vi "Quick Print VI or Documentation.vi"(6 "custom contents options":T13 {"list of controls options"."list which controls?" items=["all controls", "connected controls"]}, 7 "layout options":T1={"orientation (unchanged)"=0, "panel scaling for page (unchanged)"=0, "margins"={"override VI margins (false)"=FALSE, "margins (1.00)"={"top"=1.0, "left"=1.0, "right"=1.0, "bottom"=1.0}, "measurement system (default)"=0}, "printer options"={"destination printer name (current)"="", "printing method (unchanged)"=0, "color or monochrome (unchanged)"=0}, "page header options"={"page headers (unchanged)"=0, "page header content options"={"Include VI Name"=TRUE, "Include VI Path"=TRUE, "Include Last Modification Date"=TRUE, "Include Date Printed"=TRUE, "Include Page Number"=TRUE, "Include VI Icon"=TRUE}}} {"page header options"."page headers (unchanged)" items=["Unchanged", "Include page headers", "Do not include page headers"]; "printer options"."color or monochrome (unchanged)" items=["Unchanged", "Color/grayscale", "Monochrome"]; "printer options"."printing method (unchanged)" items=["Unchanged", "Standard", "PostScript", "Bitmap"]; "panel scaling for page (unchanged)" items=["Unchanged", "No Scaling", "Scale front panel to fit"]; "orientation (unchanged)" items=["Unchanged", "portrait", "landscape"]; "margins"."measurement system (default)" items=["Default", "US", "Metric"]; "margins"."margins (1.00)"."right" format="%.2f"; "margins"."margins (1.00)"."bottom" format="%.2f"; "margins"."margins (1.00)"."top" format="%.2f"; "margins"."margins (1.00)"."left" format="%.2f"}, 8 "error in (no error)":errorcluster, 10 "contents (complete front panel)":T15 items=["Complete front panel", "Visible portion of front panel", "Icon, description, panel and diagram", "Documentation: Using the panel", "Documentation: Using as a subVI", "Documentation: Complete", "Documentation: Custom"], 11 "VI reference":refnum<vi>) -> (0 "error out":errorcluster)   [LabVIEW 2020, in "NI_ReportGenerationCore.lvlib"]
uses:
  <vilib>/Utility/NIReport.llb/NI_ReportGenerationCore.lvlib
  <vilib>/printing/EasyPrintingControls.llb/contents.ctl
  <vilib>/printing/EasyPrintingControls.llb/custom_contents_options.ctl
  <vilib>/printing/EasyPrintingControls.llb/list_which_controls.ctl
  <vilib>/printing/EasyPrintingControls.llb/layout_options.ctl
  <vilib>/printing/EasyPrintingControls.llb/orientation.ctl
  <vilib>/printing/EasyPrintingControls.llb/panel_scaling_for_page.ctl
  <vilib>/printing/EasyPrintingControls.llb/margins.ctl
  <vilib>/printing/EasyPrintingControls.llb/margin_values.ctl
  <vilib>/printing/EasyPrintingControls.llb/measurement_system.ctl
  <vilib>/printing/EasyPrintingControls.llb/printer_options.ctl
  <vilib>/printing/EasyPrintingControls.llb/printing_method.ctl
  <vilib>/printing/EasyPrintingControls.llb/color_or_monochrome.ctl
  <vilib>/printing/EasyPrintingControls.llb/page_header_options.ctl
  <vilib>/printing/EasyPrintingControls.llb/page_headers.ctl
  <vilib>/printing/EasyPrintingControls.llb/page_header_content_options.ctl
  <vilib>/printing/EasyPrintingControls.llb/contents_ENUM.ctl
panel:
  in  "VI Type Names":string[](array[string])=["invalid VI type", "Standard VI", "Control VI", "Global VI", "Polymorphic VI"]
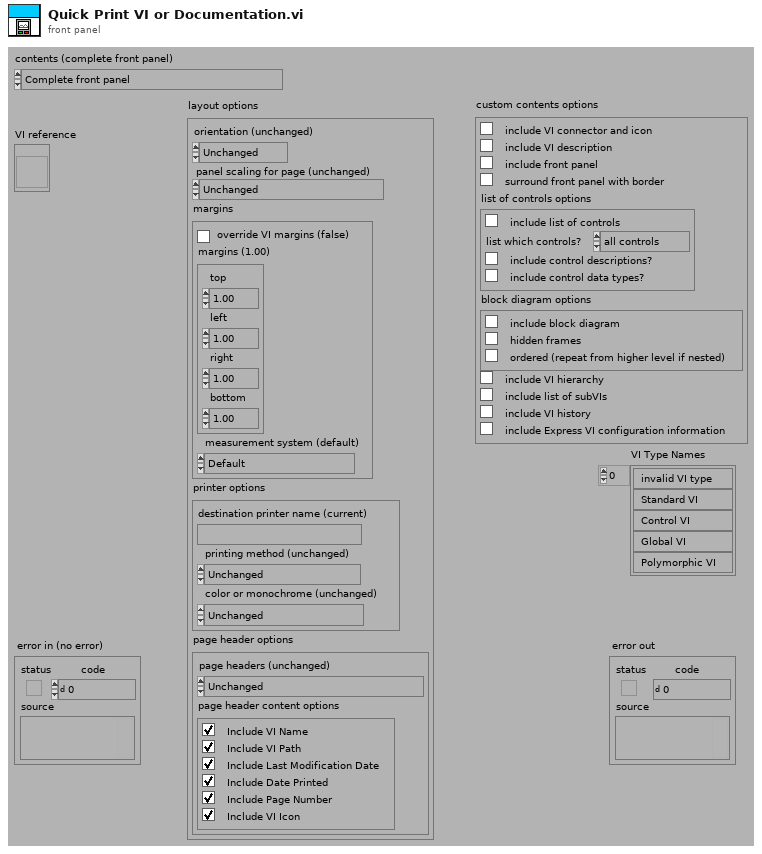
[diagram p1: front panel]
types:
  T1 = typedef "NI_ReportGenerationCore.lvlib/layout_options.ctl" = cluster{"orientation (unchanged)":T2, "panel scaling for page (unchanged)":T3, "margins":T4, "printer options":T7, "page header options":T10}
  T2 = typedef "NI_ReportGenerationCore.lvlib/orientation.ctl" = u16
  T3 = typedef "NI_ReportGenerationCore.lvlib/panel_scaling_for_page.ctl" = u16
  T4 = typedef "NI_ReportGenerationCore.lvlib/margins.ctl" = cluster{"override VI margins (false)":bool, "margins (1.00)":T5, "measurement system (default)":T6}
  T5 = typedef "NI_ReportGenerationCore.lvlib/margin_values.ctl" = cluster{"top":dbl, "left":dbl, "right":dbl, "bottom":dbl}
  T6 = typedef "NI_ReportGenerationCore.lvlib/measurement_system.ctl" = u16
  T7 = typedef "NI_ReportGenerationCore.lvlib/printer_options.ctl" = cluster{"destination printer name (current)":string, "printing method (unchanged)":T8, "color or monochrome (unchanged)":T9}
  T8 = typedef "NI_ReportGenerationCore.lvlib/printing_method.ctl" = u16
  T9 = typedef "NI_ReportGenerationCore.lvlib/color_or_monochrome.ctl" = u16
  T10 = typedef "NI_ReportGenerationCore.lvlib/page_header_options.ctl" = cluster{"page headers (unchanged)":T11, "page header content options":T12}
  T11 = typedef "NI_ReportGenerationCore.lvlib/page_headers.ctl" = u16
  T12 = typedef "NI_ReportGenerationCore.lvlib/page_header_content_options.ctl" = cluster{"Include VI Name":bool, "Include VI Path":bool, "Include Last Modification Date":bool, "Include Date Printed":bool, "Include Page Number":bool, "Include VI Icon":bool}
  T13 = typedef "NI_ReportGenerationCore.lvlib/custom_contents_options.ctl" = cluster{"include VI connector and icon":bool, "include VI description":bool, "include front panel":bool, "surround front panel with border":bool, "list of controls options":cluster{"include list of controls":bool, "list which controls?":T14, "include control descriptions?":bool, "include control data types?":bool}, "block diagram options":cluster{"include block diagram":bool, "hidden frames":bool, "ordered (repeat from higher level if nested)":bool}, "include VI hierarchy":bool, "include list of subVIs":bool, "include VI history":bool, "include Express VI configuration information":bool}
  T14 = typedef "NI_ReportGenerationCore.lvlib/list_which_controls.ctl" = u16
  T15 = typedef "NI_ReportGenerationCore.lvlib/contents.ctl" = u16
  T16 = typedef "NI_ReportGenerationCore.lvlib/contents_ENUM.ctl" = enum16{"Complete front panel", "Visible portion of front panel", "Icon, description, panel and diagram", "Documentation: Using the panel", "Documentation: Using as a subVI", "Documentation: Complete", "Documentation: Custom"}
  T17 = enum32{"invalid VI type", "Standard VI", "Control VI", "Global VI", "Polymorphic VI", "Configuration VI", "SubSystem", "Facade VI", "Method VI", "Statechart Diagram VI"}
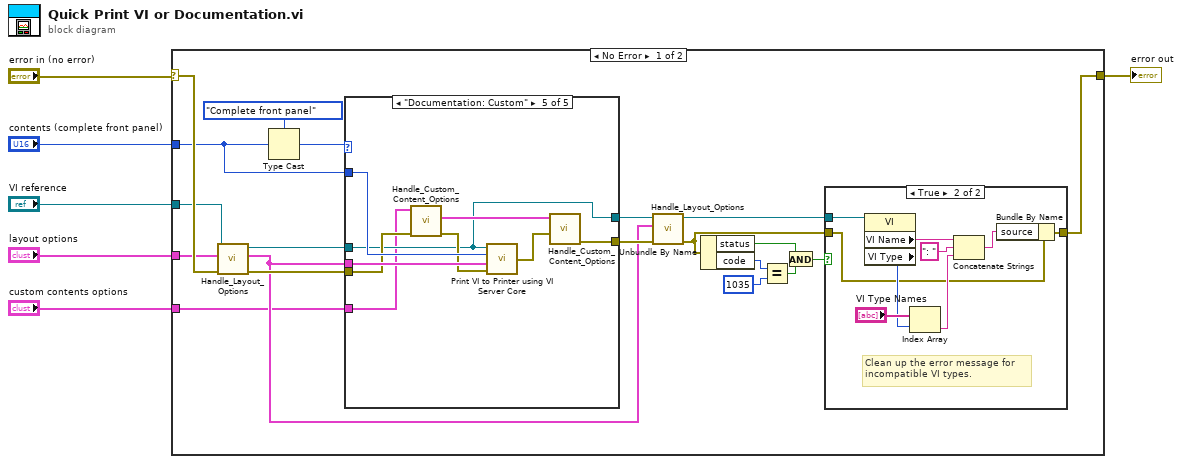
[diagram p0: block diagram]
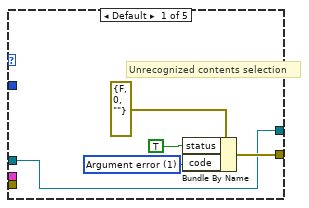
[diagram p3: hidden frame]
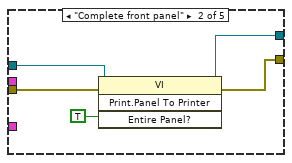
[diagram p4: hidden frame]
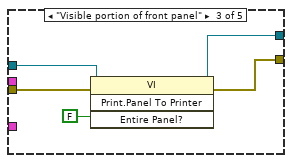
[diagram p5: hidden frame]
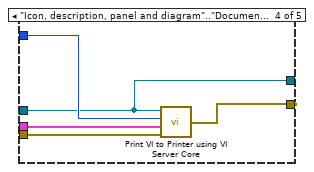
[diagram p6: hidden frame]
diagram:
  n1 = case shown="No Error" "error in (no error)" {
    selector: "error in (no error)" -> [w26 w66]
    tunnel: [w11 w66] -> w5
    tunnel: "contents (complete front panel)" -> [w10 _]
    tunnel: "layout options" -> [w9 _]
    tunnel: "custom contents options" -> [w8 _]
    tunnel: "VI reference" -> [w7 _]
    frame No Error {
      n2 = call <vilib>:"Handle_Layout_Options.vi"("error in (no error)"=w26, "layout options"=w9, "VI Refnum"=w7) -> ("error out"=w23:errorcluster, "previous layout options"=w21:T1, "VI Refnum out"=w20:refnum<vi>)  [unwired: 6 in]
      n3 = Type Cast(type=contents_ENUM."Complete front panel" ("Enum"), x=w10) -> (*(type *) &x=w24:T16)
      n4 = case shown="\"Documentation: Custom\"" w24 {
        tunnel: [w39 w44 w49 w55 w60] -> w22
        tunnel: w20 -> [w37 w43 w47 w52 w58]
        tunnel: w23 -> [_ w46 w51 w56 w63]
        tunnel: w21 -> [_ _ _ w54 w65]
        tunnel: w10 -> [_ _ _ w53 w64]
        tunnel: [w37 w42 w48 w52 w58] -> w19
        tunnel: w8 -> [_ _ _ _ w57]
        frame Default {
          w40 = 1 items=["No error", "Argument error", "Memory is full", "Out of zone", "End of file", "File already open", "Generic file I/O error", "File not found", "File permission error", "Disk is full", "Duplicate path", "Too many files open", "System feature not enabled", "Resource file not found", "Cannot add resource", "Resource not found", "Image not found", "Image memory error", "Pen does not exist", "Config type invalid", "Config token not found", "Config parse error", "Config memory error", "Bad external code format", "Bad external code offset", "External code not present", "Null window", "Destroy window error", "Null menu", "Print aborted", "Bad print record", "Print driver error", "Windows error during printing", "Memory error during printing", "Print dialog error", "Generic print error", "Invalid device refnum", "Device not found", "Device parameter error", "Device unit error", "Cannot open device", "Device call aborted", "Generic error", "Cancelled by user", "Object ID too low", "Object ID too high", "Object not in heap", "Unknown heap", "Unknown object (invalid DefProc)", "Unknown object (DefProc not in table)", "Message out of range", "Invalid (null) method", "Unknown message", "Manager call not supported", "Bad address", "Network operation in progress", "Network operation timed out", "Connection is busy", "Network attribute not supported", "Network error", "Address in use", "System out of memory", "Connection aborted", "Connection refused", "Not connected", "Already connected", "Connection closed", "Initialization error (interapplication manager)", "Bad occurrence", "Wait on unbound occurrence handler", "Occurrence queue overflow", "Datalog type conflict", "Unused", "Unrecognized type (interapplication manager)", "Memory corrupt", "Failed to make temporary DLL", "Old CIN version", "Drag socket not found", "Failed to load drop-object", "Failed to register OLE object", "Failed to release OLE object", "Format specifier type mismatch", "Unknown format specifier", "Too few format specifiers", "Too many format specifiers", "Scan failed", "Newer CIN version", "Error converting to variant", "Runtime menu error", "Password tampered", "Variant attribute not found", "Incompatible variant data type", "Event data is not available", "Event Store is not present", "Occurrence is not found", "Event Queue is not created", "Event info is not available", "Refnum passed is NULL", "Error retrieving Class GUID", "Error retrieving CoClass GUID", "Error retrieving TypeLib GUID.", "Bad built application magic bytes.", "Specific driver is different from the specific driver associated with the Logical Name.", "There is no session opened to the class driver.", "Max Error", "MAX - Error with config objects", "MAX - Error loading configuration", "MAX - Group not supported"]
          # "Unrecognized contents selection"
          n5 = Bundle By Name(cluster=errorcluster {"status"=FALSE, "code"=0, "source"=""} ("error IO"), "status"=TRUE, "code"=w40) -> (w39:errorcluster)
        }
        frame "Complete front panel" {
          n6 = invoke class="VI" method="Print.Panel To Printer"(reference=w43, error in=w46, "Entire Panel?"=TRUE) -> (reference out=w42:refnum<vi>, error out=w44:errorcluster)  [unwired: 1 in, 2 out]
        }
        frame "Visible portion of front panel" {
          n7 = invoke class="VI" method="Print.Panel To Printer"(reference=w47, error in=w51, "Entire Panel?"=FALSE) -> (reference out=w48:refnum<vi>, error out=w49:errorcluster)  [unwired: 1 in, 2 out]
        }
        frame "Icon, description, panel and diagram".."Documentation: Complete" {
          n8 = call <vilib>:"Print VI to Printer using VI Server Core.vi"("error in"=w56, "layout options"=w54, "Format"=w53, "VI reference"=w52) -> ("error out"=w55:errorcluster)
        }
        frame "Documentation: Custom" {
          n9 = call <vilib>:"Handle_Custom_Content_Options.vi"("error in (no error)"=w63, "custom contents options"=w57) -> ("error out"=w62:errorcluster, "previous custom contents options"=w59:T13)  [unwired: 8 in]
          n10 = call <vilib>:"Print VI to Printer using VI Server Core.vi"("error in"=w62, "layout options"=w65, "Format"=w64, "VI reference"=w58) -> ("error out"=w61:errorcluster)
          n11 = call <vilib>:"Handle_Custom_Content_Options.vi"("error in (no error)"=w61, "custom contents options"=w59) -> ("error out"=w60:errorcluster)  [unwired: 8 in, 1 out]
        }
      }
      n12 = call <vilib>:"Handle_Layout_Options.vi"("error in (no error)"=w22, "layout options"=w21, "VI Refnum"=w19) -> ("error out"=w12:errorcluster, "VI Refnum out"=w14:refnum<vi>)  [unwired: 6 in, 1 out]
      n13 = Unbundle By Name(w12) -> ("status"=w15:bool, "code"=w18:i32)
      n14 = Equal?(x=w18, y=1035 ("code")) -> (x = y?=w16:bool)
      n15 = And(x=w15, y=w16) -> (x .and. y?=w13:bool)
      n16 = case shown="True" w13 {
        tunnel: w14 -> [_ w36]
        tunnel: [w27 w28] -> w11
        tunnel: w12 -> [w27 w30]
        frame False {
        }
        frame True {
          # "Clean up the error message for \nincompatible VI types."
          n17 = property class="VI"(reference=w36) -> ("VI Name"=w33:string, "VI Type"=w34:T17)  [unwired: 1 in, 2 out]
          n18 = Index Array(array="VI Type Names", index=w34) -> (element=w32:string)
          n19 = Concatenate Strings(w33, ": " ("string"), w32) -> (w29:string)
          n20 = Bundle By Name(cluster=w30, "source"=w29) -> (w28:errorcluster)
        }
      }
    }
    frame Error {
    }
  }
  "error out" <- w5
